vi "Z900_navX_Internal_StartLoop.vi"(8 "error in (no error)":errorcluster, 11 "navX Device":T1={"Interface"={"Protocol"=enum."SERIAL", "Update Rate (4Hz-60Hz)"=4, "navX Open TypeDef"=variant}, "Notify Packet"=refnum, "Loop VI Refnum"=refnum, "Ready to Close Occurrence Refnum"=refnum} {"Interface"."Update Rate (4Hz-60Hz)" min=4 max=60 step=1}) -> (0 "error out":errorcluster, 3 "navX Device":T1={"Interface"={"Protocol"=enum."SERIAL", "Update Rate (4Hz-60Hz)"=4, "navX Open TypeDef"=variant}, "Notify Packet"=refnum, "Loop VI Refnum"=refnum, "Ready to Close Occurrence Refnum"=refnum} {"Interface"."Update Rate (4Hz-60Hz)" min=4 max=60 step=1})   [LabVIEW 2015, in "navX Library v2.lvlib"]
doc: "This navX VI handles starting the background processing loop for the navX.\nTHIS VI SHOULD NOT BE CALLED BY THE USER!"
uses:
  navX Library v2.lvlib
  TypeDefs/Z900_navX_DeviceTypeDef.ctl
  TypeDefs/Z900_navX_ProtocolTypeDef.ctl
  TypeDefs/Z900_navX_NotifyPacketTypeDef.ctl
  TypeDefs/Z900_navX_ActionTypeDef.ctl
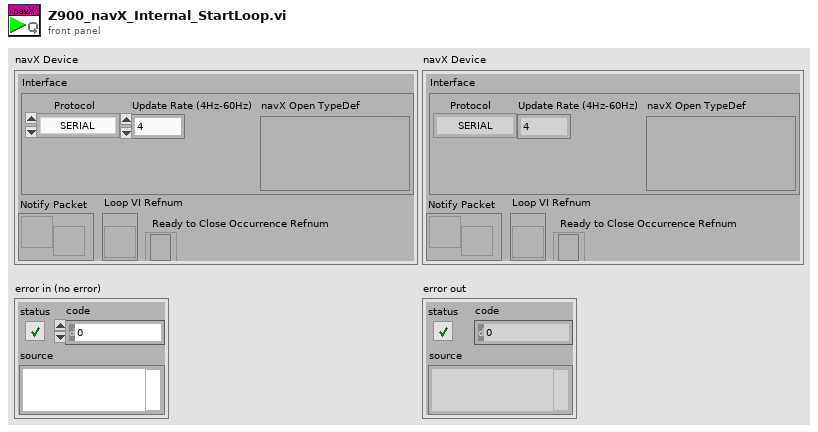
[diagram p1: front panel]
types:
  T1 = typedef "navX Library v2.lvlib/Z900_navX_DeviceTypeDef.ctl" = cluster{"Interface":cluster{"Protocol":T2, "Update Rate (4Hz-60Hz)":u8, "navX Open TypeDef":variant}, "Notify Packet":refnum<notifier>, "Loop VI Refnum":refnum<vi>, "Ready to Close Occurrence Refnum":refnum<k4>}
  T2 = typedef "navX Library v2.lvlib/Z900_navX_ProtocolTypeDef.ctl" = enum16{"SERIAL", "I2C", "SPI"}
  T3 = typedef "navX Library v2.lvlib/Z900_navX_NotifyPacketTypeDef.ctl" = cluster{"navX Action":T4, "Data":variant}
  T4 = typedef "navX Library v2.lvlib/Z900_navX_ActionTypeDef.ctl" = enum16{"None", "Halt", "Zero-Yaw", "Update Serial Protocol"}
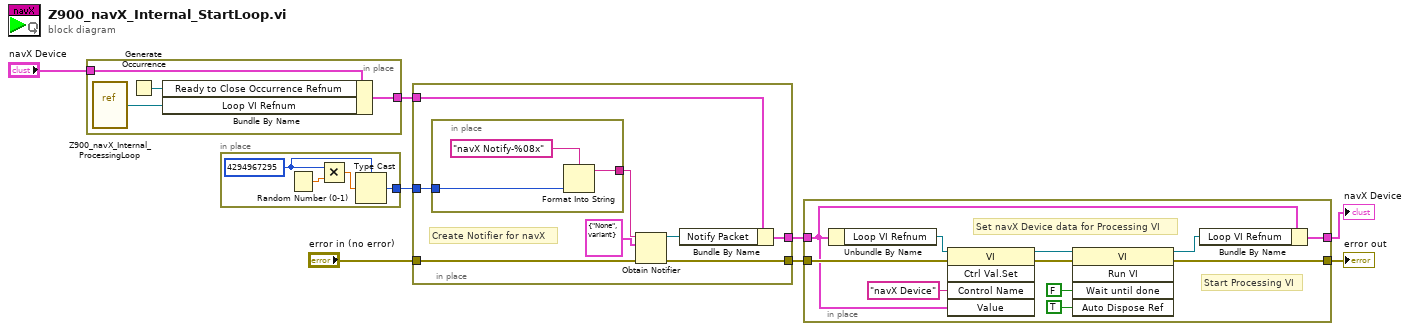
[diagram p0: block diagram]
diagram:
  n1 = in-place {
    in-place-border: "navX Device" -> [w12]
    in-place-border: [w10] -> w1
    n2 = vi-ref "Z900_navX_Internal_ProcessingLoop.vi"() -> (w9:refnum<vi>)
    n3 = Generate Occurrence() -> (w11:refnum<k4>)
    n4 = Bundle By Name(cluster=w12, "Ready to Close Occurrence Refnum"=w11, "Loop VI Refnum"=w9) -> (w10:T1)
  }
  n5 = in-place {
    in-place-border: [w13] -> w8
    w15 = u32 4294967295
    n6 = Random Number (0-1)() -> (number: 0 to 1=w16:dbl)
    n7 = Multiply(x=w15, y=w16) -> (x*y=w14:dbl)
    n8 = Type Cast(type=w15, x=w14) -> (*(type *) &x=w13:u32)
  }
  n9 = in-place {
    in-place-border: w1 -> [w24]
    in-place-border: [w23] -> w5
    in-place-border: "error in (no error)" -> [w20]
    in-place-border: w8 -> [w18]
    in-place-border: [w17] -> w6
    # "Create Notifier for navX"
    n10 = in-place {
      in-place-border: [w26] -> w19
      in-place-border: w18 -> [w25]
      n11 = Format Into String(format string="navX Notify-%08x" ("name (unnamed)"), w25) -> (resulting string=w26:string)  [unwired: 2 in, 1 out]
    }
    n12 = Obtain Notifier(name (unnamed)=w19, notification data type=T3 {"navX Action"=enum."None", "Data"=variant} ("navX Notify Packet"), error in (no error)=w20) -> (notifier out=w22:refnum<notifier>, error out=w17:errorcluster)  [unwired: 1 in, 1 out]
    n13 = Bundle By Name(cluster=w24, "Notify Packet"=w22) -> (w23:T1)
  }
  n14 = in-place {
    in-place-border: w6 -> [w30]
    in-place-border: [w37] -> w4
    in-place-border: [w38] -> w3
    in-place-border: w5 -> [w29]
    # "Start Processing VI"
    # "Set navX Device data for Processing VI"
    n15 = Unbundle By Name(w29) -> ("Loop VI Refnum"=w28:refnum<vi>)
    n16 = invoke class="VI" method="Ctrl Val.Set"(reference=w28, error in=w30, "Control Name"="navX Device" ("format string"), "Value"=w29) -> (reference out=w33:refnum<vi>, error out=w32:errorcluster)  [unwired: 1 in, 3 out]
    n17 = invoke class="VI" method="Run VI"(reference=w33, error in=w32, "Wait until done"=FALSE ("Wait Until Done"), "Auto Dispose Ref"=TRUE ("Auto Dispose Reference")) -> (reference out=w31:refnum<vi>, error out=w38:errorcluster)  [unwired: 1 in, 3 out]
    n18 = Bundle By Name(cluster=w29, "Loop VI Refnum"=w31) -> (w37:T1)
  }
  "navX Device" <- w4
  "error out" <- w3
